vi "MQTT_PubRec_Send.vi"(8 "error in (no error)":errorcluster, 10 "Message ID":u16=10 format="%x", 11 "SSL_Connection":T1) -> (0 "error out":errorcluster, 2 "PubRec Message":u8[](array[numeric]) format="%x", 3 "SSL_Connection 2":T1)   [LabVIEW 2015]
uses:
  Controls/SSL_Connection.ctl
  Controls/Retain_Flag.ctl
  Controls/MessageType.ctl
  Controls/DUP_Flag.ctl
  Controls/QoS.ctl
  AWS_IoT.lvlib
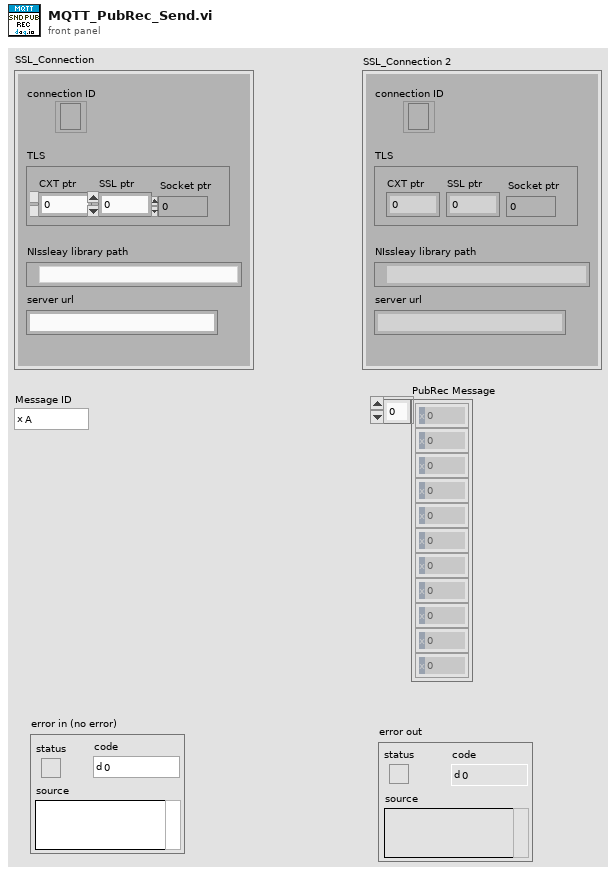
[diagram p1: front panel]
types:
  T1 = typedef "AWS_IoT.lvlib/SSL_Connection.ctl" = cluster{"connection ID":refnum<k5>, "TLS":cluster{"CXT ptr":i32, "SSL ptr":i32, "Socket ptr":i32}, "NIssleay library path":path, "server url":string}
  T2 = typedef "QoS.ctl" = enum8{"At most once", "At least once", "Exactly once", "Reserved"}
  T3 = typedef "DUP_Flag.ctl" = bool
  T4 = typedef "MessageType.ctl" = enum32{"Reserved", "CONNECT", "CONNACK", "PUBLISH", "PUBACK", "PUBREC", "PUBREL", "PUBCOMP", "SUBSCRIBE", "SUBACK", "UNSUBSCRIBE", "UNSUBACK", "PINGREQ", "PINGRESP", "DISCONNECT", "Reserved2"}
  T5 = typedef "Retain_Flag.ctl" = bool
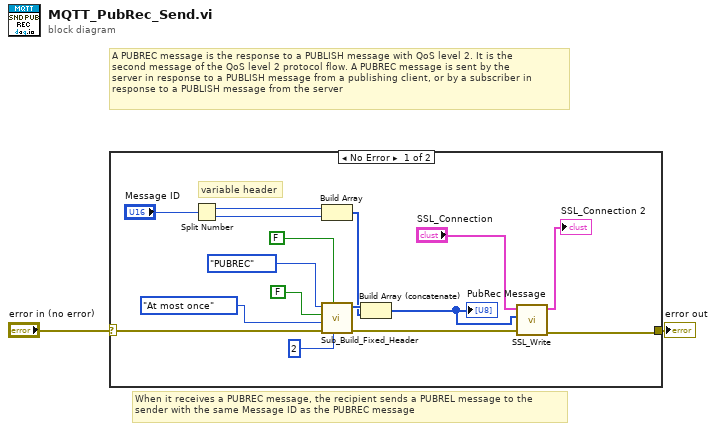
[diagram p0: block diagram]
diagram:
  # "When it receives a PUBREC message, the recipient sends a PUBREL message to the\nsender with the same Message ID as the PUBREC message"
  # "A PUBREC message is the response to a PUBLISH message with QoS level 2. It is the\nsecond message of the QoS level 2 protocol flow. A PUBREC message is sent by the\nserver in response to a PUBLISH message from a publishing client, or by a subscriber in\nresponse to a PUBLISH message from the server"
  n1 = case shown="No Error" "error in (no error)" {
    selector: "error in (no error)" -> [w13 w19]
    tunnel: [w9 w19] -> w1
    frame No Error {
      # "variable header"
      n2 = Split Number(x="Message ID") -> (hi(x)=w17:u8, lo(x)=w16:u8)
      n3 = Build Array(w17, w16) -> (w12:u8[])
      n4 = call "Sub_Build_Fixed_Header.vi"("Remaining Length"=u32 2, "Retain"=T5 FALSE, "error in (no error)"=w13, "QoS"=QoS."At most once", "DUP"=T3 FALSE, "MessageType"=MessageType."PUBREC") -> ("error out"=w10:errorcluster, "Fixed Header"=w18:u8[])  [unwired: 4 in]
      n5 = Build Array (concatenate)(w18, w12) -> (w11:u8[])
      "PubRec Message" <- w11
      n6 = call "SSL_Write.vi"("error in (no error)"=w10, "data in"=w11, "SSL_Connection"="SSL_Connection") -> ("error out"=w9:errorcluster, "SSL_Connection"=→"SSL_Connection 2":T1)  [unwired: 7 in]
    }
    frame Error {
    }
  }
  "error out" <- w1
